vi "Create Client.vi"(8 "error in":errorcluster, 10 "Server Certificate File (.crt)":path, 11 "address":string) -> (0 "error out":errorcluster, 3 "gRPC ID Out":T1)   [LabVIEW 2021, in "Template_Wrapper.lvlib"]
uses:
  Template_Wrapper.lvlib
  <vilib>/gRPC/LabVIEW gRPC Library/Shared/grpcId.ctl
  <vilib>/gRPC/LabVIEW gRPC Library/grpc-lvsupport-release.lvlib
  <vilib>/CIF Foundation/CIF Core/CIFUtilities/CIFConfigurationFile/CIF Configuration File.lvlib
  Template_client/Template_client.lvlib
  <vilib>/CIF Foundation/CIF Core/CIFCore/Grpc/CIFCorePlugin_client/CIFCorePlugin_client.lvlib
  <vilib>/CIF Foundation/CIF Core/CIFCore/Grpc/CIFCoreChannel_client/CIFCoreChannel_client.lvlib
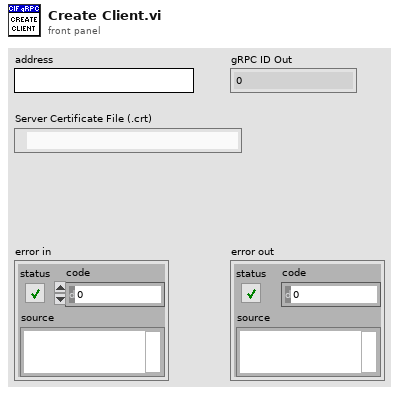
[diagram p1: front panel]
types:
  T1 = typedef "grpc-lvsupport-release.lvlib/grpcId.ctl" = u64
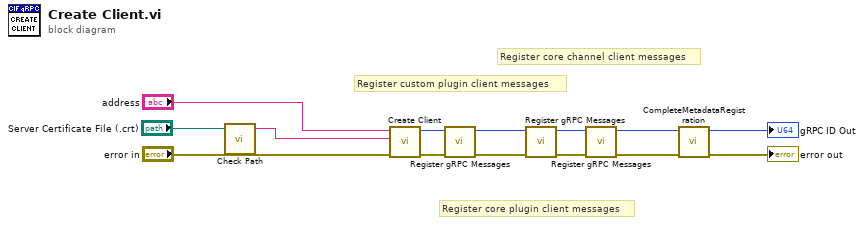
[diagram p0: block diagram]
diagram:
  # "Register core channel client messages"
  # "Register core plugin client messages"
  # "Register custom plugin client messages"
  n1 = call <vilib>:"Check Path.vi"("path"="Server Certificate File (.crt)") -> ("Path String"=w7:string)  [unwired: 3 in]
  n2 = call <vilib>:"Create Client.vi"("error in"="error in", "certificatePath"=w7, "address"="address") -> ("error out"=w9:errorcluster, "ClientID out"=w10:T1)  [unwired: 7 in]
  n3 = call <vilib>:"Register gRPC Messages.vi"("error in (no error)"=w9, "gRPC ID"=w10) -> ("error out"=w3:errorcluster, "gRPC ID Out"=w4:T1)  [unwired: 8 in]
  n4 = call <vilib>:"Register gRPC Messages.vi"("error in (no error)"=w3, "gRPC ID"=w4) -> ("error out"=w6:errorcluster, "gRPC ID Out"=w5:T1)  [unwired: 8 in]
  n5 = call <vilib>:"Register gRPC Messages.vi"("error in (no error)"=w6, "gRPC ID"=w5) -> ("error out"=w1:errorcluster, "gRPC ID Out"=w2:T1)  [unwired: 8 in]
  n6 = call <vilib>:"CompleteMetadataRegistration.vi"("error in"=w1, "gRPC ID in"=w2) -> ("error out"=→"error out":errorcluster, "gRPC ID Out"=→"gRPC ID Out":T1)  [unwired: 8 in]
